vi "RGB_MNIST_PMT_sub.vi"(1 "pixel size":sgl=3.1, 2 "B_2D(28x28)":i32[][](array[numeric])=[[0, 0, 0, 0, 0, 0, 0, 0, 0, 0, 0, 0, 0, 0, 0, 0, 0, 0, 0, 0, 0, 0, 0, 0, 0, 0, 0, 0], [0, 0, 0, 0, 0, 0, 0, 0, 0, 0, 0, 1, 0, 0, 0, 0, 0, 0, 0, 0, 0, 0, 0, 0, 0, 0, 0, 0], [0, 0, 0, 0, 0, 0, 0, 0, 0, 0, 0, 3, 2, 0, 0, 0, 0, 0, 0, 0, 0, 0, 0, 0, 0, 0, 0, 0], [0, 0, 0, 0, 0, 0, 0, 6, 23, 26, 13, 4, 1, 0, 9, 27, 34, 24, 5, 0, 0, 0, 0, 0, 0, 0, 0, 0], [0, 0, 0, 0, 0, 0, 15, 47, 55, 55, 51, 40, 9, 7, 46, 57, 50, 16, 1, 0, 0, 0, 0, 0, 0, 0, 0, 0], [0, 0, 0, 0, 0, 12, 50, 57, 55, 57, 60, 63, 30, 30, 62, 82, 84, 72, 54, 20, 2, 0, 0, 0, 0, 0, 0, 0], [0, 0, 0, 0, 4, 44, 56, 54, 66, 89, 117, 131, 124, 100, 123, 137, 137, 138, 140, 138, 90, 26, 0, 0, 0, 0, 0, 0], [0, 0, 0, 0, 29, 55, 60, 91, 126, 139, 137, 136, 136, 136, 134, 133, 136, 137, 140, 142, 147, 131, 46, 0, 0, 0, 0, 0], [0, 0, 0, 10, 47, 62, 110, 151, 149, 145, 143, 143, 142, 139, 138, 136, 135, 137, 141, 144, 146, 150, 137, 36, 0, 0, 0, 0], [0, 0, 0, 27, 47, 104, 163, 161, 156, 155, 152, 150, 149, 146, 145, 140, 136, 137, 142, 144, 146, 150, 157, 109, 3, 0, 0, 0], [0, 0, 4, 14, 29, 139, 174, 168, 162, 162, 160, 158, 154, 153, 151, 144, 139, 138, 143, 144, 145, 148, 156, 141, 46, 0, 0, 0], [0, 0, 0, 0, 60, 167, 176, 170, 166, 165, 164, 162, 160, 156, 153, 150, 143, 140, 143, 144, 145, 147, 154, 155, 82, 0, 0, 0], [0, 0, 0, 0, 89, 185, 184, 175, 172, 168, 165, 163, 164, 161, 157, 153, 147, 142, 143, 144, 144, 146, 153, 160, 101, 0, 0, 0], [0, 0, 0, 0, 93, 191, 188, 180, 176, 170, 167, 168, 169, 165, 161, 156, 150, 143, 143, 144, 145, 147, 153, 159, 109, 6, 0, 0], [0, 0, 0, 0, 84, 186, 191, 185, 179, 173, 170, 170, 169, 166, 162, 157, 151, 144, 143, 144, 145, 148, 153, 159, 112, 11, 0, 0], [0, 0, 0, 0, 60, 178, 196, 190, 182, 176, 172, 171, 170, 167, 162, 157, 151, 144, 143, 144, 145, 149, 153, 159, 107, 4, 0, 0], [0, 0, 0, 0, 18, 165, 204, 193, 184, 177, 174, 171, 170, 167, 161, 158, 152, 143, 142, 144, 145, 149, 153, 159, 94, 0, 0, 0], [0, 0, 0, 0, 0, 121, 202, 195, 186, 179, 175, 171, 169, 167, 162, 158, 153, 144, 141, 144, 145, 149, 154, 150, 72, 0, 0, 0], [0, 0, 0, 0, 0, 38, 181, 200, 190, 181, 175, 172, 168, 166, 160, 158, 151, 142, 141, 144, 146, 149, 157, 135, 30, 0, 0, 0], [0, 0, 0, 0, 0, 0, 101, 204, 193, 182, 177, 172, 168, 165, 159, 157, 148, 138, 140, 144, 147, 149, 154, 90, 0, 0, 0, 0], [0, 0, 0, 0, 0, 0, 10, 121, 196, 184, 178, 171, 167, 162, 159, 156, 144, 137, 141, 143, 146, 149, 104, 14, 0, 0, 0, 0], [0, 0, 0, 0, 0, 0, 0, 11, 91, 176, 178, 171, 162, 157, 156, 148, 139, 138, 142, 145, 143, 86, 13, 0, 0, 0, 0, 0], [0, 0, 0, 0, 0, 0, 0, 0, 0, 41, 127, 162, 158, 152, 146, 141, 138, 138, 136, 116, 45, 2, 0, 0, 0, 0, 0, 0], [0, 0, 0, 0, 0, 0, 0, 0, 0, 0, 4, 49, 98, 121, 133, 144, 147, 121, 49, 5, 0, 0, 0, 0, 0, 0, 0, 0], [0, 0, 0, 0, 0, 0, 0, 0, 0, 0, 0, 0, 0, 17, 52, 83, 101, 55, 0, 0, 0, 0, 0, 0, 0, 0, 0, 0], [0, 0, 0, 0, 0, 0, 0, 0, 0, 0, 0, 0, 0, 0, 0, 1, 4, 2, 0, 0, 0, 0, 0, 0, 0, 0, 0, 0], [0, 0, 0, 0, 0, 0, 0, 0, 0, 0, 0, 0, 0, 0, 0, 0, 0, 0, 0, 0, 0, 0, 0, 0, 0, 0, 0, 0], [0, 0, 0, 0, 0, 0, 0, 0, 0, 0, 0, 0, 0, 0, 0, 0, 0, 0, 0, 0, 0, 0, 0, 0, 0, 0, 0, 0], [255, 0, 0, 0, 0, 0, 0, 0, 0, 0, 0, 0, 0, 0, 0, 0, 0, 0, 0, 0, 0, 0, 0, 0, 0, 0, 0, 0]], 3 "G_2D(28x28)":i32[][](array[numeric])=[[0, 0, 0, 0, 0, 0, 0, 0, 0, 0, 0, 0, 0, 0, 0, 0, 0, 0, 0, 0, 0, 0, 0, 0, 0, 0, 0, 0], [0, 0, 0, 0, 0, 0, 0, 0, 0, 0, 0, 1, 1, 0, 0, 0, 0, 0, 0, 0, 0, 0, 0, 0, 0, 0, 0, 0], [0, 0, 0, 0, 0, 0, 0, 0, 0, 0, 0, 6, 4, 0, 0, 0, 0, 0, 0, 0, 0, 0, 0, 0, 0, 0, 0, 0], [0, 0, 0, 0, 0, 0, 0, 13, 47, 51, 26, 8, 3, 0, 18, 54, 65, 45, 7, 0, 0, 0, 0, 0, 0, 0, 0, 0], [0, 0, 0, 0, 0, 0, 28, 90, 107, 109, 101, 75, 15, 14, 91, 112, 96, 30, 1, 0, 0, 0, 0, 0, 0, 0, 0, 0], [0, 0, 0, 0, 0, 23, 97, 113, 111, 110, 113, 117, 50, 55, 111, 117, 96, 71, 54, 20, 2, 0, 0, 0, 0, 0, 0, 0], [0, 0, 0, 0, 8, 85, 112, 109, 112, 119, 128, 132, 126, 112, 128, 137, 137, 138, 140, 138, 90, 26, 0, 0, 0, 0, 0, 0], [0, 0, 0, 0, 56, 109, 112, 122, 133, 137, 137, 136, 136, 136, 133, 134, 136, 137, 139, 142, 147, 131, 46, 0, 0, 0, 0, 0], [0, 0, 0, 18, 92, 116, 133, 149, 149, 145, 143, 143, 142, 139, 138, 136, 135, 137, 141, 143, 146, 150, 137, 36, 0, 0, 0, 0], [0, 0, 0, 53, 97, 128, 163, 161, 156, 155, 152, 150, 149, 146, 145, 141, 137, 137, 142, 144, 146, 150, 157, 109, 3, 0, 0, 0], [0, 0, 7, 28, 38, 140, 173, 168, 162, 162, 160, 158, 154, 153, 150, 144, 139, 138, 143, 144, 145, 148, 156, 141, 46, 0, 0, 0], [0, 0, 0, 0, 60, 167, 175, 170, 166, 165, 164, 162, 160, 156, 153, 150, 143, 140, 143, 144, 145, 148, 154, 155, 82, 0, 0, 0], [0, 0, 0, 0, 88, 184, 184, 176, 172, 168, 165, 163, 164, 161, 157, 153, 147, 142, 143, 144, 144, 147, 153, 160, 101, 0, 0, 0], [0, 0, 0, 0, 93, 190, 188, 180, 176, 171, 167, 168, 169, 165, 161, 156, 150, 143, 143, 144, 144, 147, 153, 159, 109, 6, 0, 0], [0, 0, 0, 0, 84, 186, 191, 185, 179, 173, 170, 170, 169, 166, 162, 157, 151, 144, 143, 144, 145, 148, 153, 159, 112, 11, 0, 0], [0, 0, 0, 0, 60, 177, 196, 190, 182, 176, 172, 171, 170, 167, 162, 157, 151, 144, 143, 144, 145, 149, 153, 159, 107, 4, 0, 0], [0, 0, 0, 0, 18, 165, 204, 193, 184, 177, 173, 171, 170, 167, 161, 158, 152, 145, 142, 144, 145, 149, 153, 159, 94, 0, 0, 0], [0, 0, 0, 0, 0, 121, 202, 195, 185, 178, 175, 172, 170, 167, 163, 159, 153, 144, 141, 144, 145, 150, 154, 150, 72, 0, 0, 0], [0, 0, 0, 0, 0, 38, 182, 200, 190, 181, 175, 172, 168, 166, 161, 159, 152, 142, 141, 144, 146, 149, 157, 135, 30, 0, 0, 0], [0, 0, 0, 0, 0, 0, 101, 204, 192, 182, 177, 172, 168, 165, 159, 158, 148, 138, 140, 144, 147, 149, 154, 90, 0, 0, 0, 0], [0, 0, 0, 0, 0, 0, 10, 122, 196, 184, 178, 171, 167, 162, 159, 156, 144, 137, 141, 143, 146, 149, 104, 14, 0, 0, 0, 0], [0, 0, 0, 0, 0, 0, 0, 11, 91, 176, 178, 169, 162, 157, 156, 148, 139, 139, 142, 144, 143, 86, 13, 0, 0, 0, 0, 0], [0, 0, 0, 0, 0, 0, 0, 0, 0, 42, 127, 162, 158, 152, 146, 141, 138, 138, 136, 116, 45, 2, 0, 0, 0, 0, 0, 0], [0, 0, 0, 0, 0, 0, 0, 0, 0, 0, 4, 50, 98, 121, 134, 144, 147, 121, 49, 5, 0, 0, 0, 0, 0, 0, 0, 0], [0, 0, 0, 0, 0, 0, 0, 0, 0, 0, 0, 0, 0, 17, 52, 83, 101, 55, 0, 0, 0, 0, 0, 0, 0, 0, 0, 0], [0, 0, 0, 0, 0, 0, 0, 0, 0, 0, 0, 0, 0, 0, 0, 1, 4, 2, 0, 0, 0, 0, 0, 0, 0, 0, 0, 0], [0, 0, 0, 0, 0, 0, 0, 0, 0, 0, 0, 0, 0, 0, 0, 0, 0, 0, 0, 0, 0, 0, 0, 0, 0, 0, 0, 0], [0, 0, 0, 0, 0, 0, 0, 0, 0, 0, 0, 0, 0, 0, 0, 0, 0, 0, 0, 0, 0, 0, 0, 0, 0, 0, 0, 0], [255, 0, 0, 0, 0, 0, 0, 0, 0, 0, 0, 0, 0, 0, 0, 0, 0, 0, 0, 0, 0, 0, 0, 0, 0, 0, 0, 0]], 4 "R_2D(28x28)":i32[][](array[numeric])=[[0, 0, 0, 0, 0, 0, 0, 0, 0, 0, 0, 0, 0, 0, 0, 0, 0, 0, 0, 0, 0, 0, 0, 0, 0, 0, 0, 0], [0, 0, 0, 0, 0, 0, 0, 0, 0, 0, 0, 3, 1, 0, 0, 0, 0, 0, 0, 0, 0, 0, 0, 0, 0, 0, 0, 0], [0, 0, 0, 0, 0, 0, 0, 0, 0, 0, 0, 14, 9, 0, 0, 0, 0, 0, 0, 0, 0, 0, 0, 0, 0, 0, 0, 0], [0, 0, 0, 0, 0, 0, 0, 12, 44, 49, 23, 15, 8, 0, 17, 51, 61, 42, 7, 0, 0, 0, 0, 0, 0, 0, 0, 0], [0, 0, 0, 0, 0, 0, 26, 84, 100, 102, 93, 73, 19, 13, 85, 104, 89, 27, 1, 0, 0, 0, 0, 0, 0, 0, 0, 0], [0, 0, 0, 0, 0, 21, 91, 106, 102, 104, 110, 115, 61, 55, 112, 147, 148, 128, 95, 35, 4, 0, 0, 0, 0, 0, 0, 0], [0, 0, 0, 0, 9, 80, 104, 102, 123, 166, 213, 237, 229, 181, 220, 244, 245, 247, 249, 241, 159, 45, 0, 0, 0, 0, 0, 0], [0, 0, 0, 0, 54, 100, 109, 163, 226, 250, 247, 245, 245, 248, 244, 243, 245, 245, 246, 249, 255, 226, 78, 0, 0, 0, 0, 0], [0, 0, 0, 18, 86, 112, 189, 252, 252, 249, 249, 250, 248, 247, 246, 245, 244, 246, 247, 249, 251, 255, 228, 60, 0, 0, 0, 0], [0, 0, 0, 50, 87, 171, 252, 255, 252, 253, 252, 252, 253, 251, 250, 248, 244, 245, 249, 250, 251, 253, 255, 182, 4, 0, 0, 0], [0, 0, 7, 26, 47, 212, 255, 255, 255, 254, 254, 254, 254, 255, 254, 251, 247, 246, 249, 250, 250, 252, 255, 232, 75, 0, 0, 0], [0, 0, 0, 0, 87, 237, 255, 255, 255, 254, 255, 254, 254, 255, 255, 253, 249, 248, 249, 250, 251, 252, 255, 255, 136, 0, 0, 0], [0, 0, 0, 0, 124, 252, 255, 255, 254, 254, 255, 255, 254, 255, 255, 255, 252, 248, 249, 250, 251, 251, 255, 255, 167, 0, 0, 0], [0, 0, 0, 0, 124, 252, 254, 254, 255, 255, 255, 255, 255, 254, 255, 255, 252, 247, 250, 250, 251, 252, 255, 255, 180, 10, 0, 0], [0, 0, 0, 0, 106, 241, 253, 254, 255, 255, 255, 255, 255, 255, 255, 253, 249, 248, 250, 250, 250, 253, 255, 255, 188, 19, 0, 0], [0, 0, 0, 0, 76, 228, 255, 255, 255, 255, 255, 255, 255, 255, 254, 250, 250, 250, 250, 250, 251, 253, 255, 255, 178, 7, 0, 0], [0, 0, 0, 0, 23, 208, 255, 255, 255, 255, 255, 255, 255, 254, 251, 253, 253, 249, 248, 250, 251, 253, 255, 255, 156, 0, 0, 0], [0, 0, 0, 0, 0, 152, 255, 255, 254, 255, 255, 255, 255, 254, 255, 255, 254, 249, 247, 250, 251, 254, 255, 250, 118, 0, 0, 0], [0, 0, 0, 0, 0, 48, 229, 255, 254, 254, 255, 255, 254, 255, 255, 255, 254, 248, 247, 249, 251, 253, 255, 221, 49, 0, 0, 0], [0, 0, 0, 0, 0, 0, 127, 253, 255, 254, 255, 254, 255, 255, 255, 255, 253, 246, 247, 250, 252, 253, 254, 150, 0, 0, 0, 0], [0, 0, 0, 0, 0, 0, 14, 154, 255, 255, 254, 255, 255, 255, 255, 255, 250, 245, 248, 249, 251, 255, 177, 23, 0, 0, 0, 0], [0, 0, 0, 0, 0, 0, 0, 13, 124, 245, 255, 255, 254, 255, 254, 251, 246, 247, 249, 250, 248, 149, 23, 0, 0, 0, 0, 0], [0, 0, 0, 0, 0, 0, 0, 0, 1, 60, 190, 250, 255, 255, 252, 248, 246, 246, 242, 202, 78, 5, 0, 0, 0, 0, 0, 0], [0, 0, 0, 0, 0, 0, 0, 0, 0, 0, 7, 80, 166, 211, 235, 254, 255, 215, 86, 8, 0, 0, 0, 0, 0, 0, 0, 0], [0, 0, 0, 0, 0, 0, 0, 0, 0, 0, 0, 0, 0, 29, 90, 146, 177, 95, 0, 0, 0, 0, 0, 0, 0, 0, 0, 0], [0, 0, 0, 0, 0, 0, 0, 0, 0, 0, 0, 0, 0, 0, 0, 1, 7, 2, 0, 0, 0, 0, 0, 0, 0, 0, 0, 0], [0, 0, 0, 0, 0, 0, 0, 0, 0, 0, 0, 0, 0, 0, 0, 0, 0, 0, 0, 0, 0, 0, 0, 0, 0, 0, 0, 0], [0, 0, 0, 0, 0, 0, 0, 0, 0, 0, 0, 0, 0, 0, 0, 0, 0, 0, 0, 0, 0, 0, 0, 0, 0, 0, 0, 0], [255, 0, 0, 0, 0, 0, 0, 0, 0, 0, 0, 0, 0, 0, 0, 0, 0, 0, 0, 0, 0, 0, 0, 0, 0, 0, 0, 0]]) -> (0 "picture":picture)   [LabVIEW 2021]
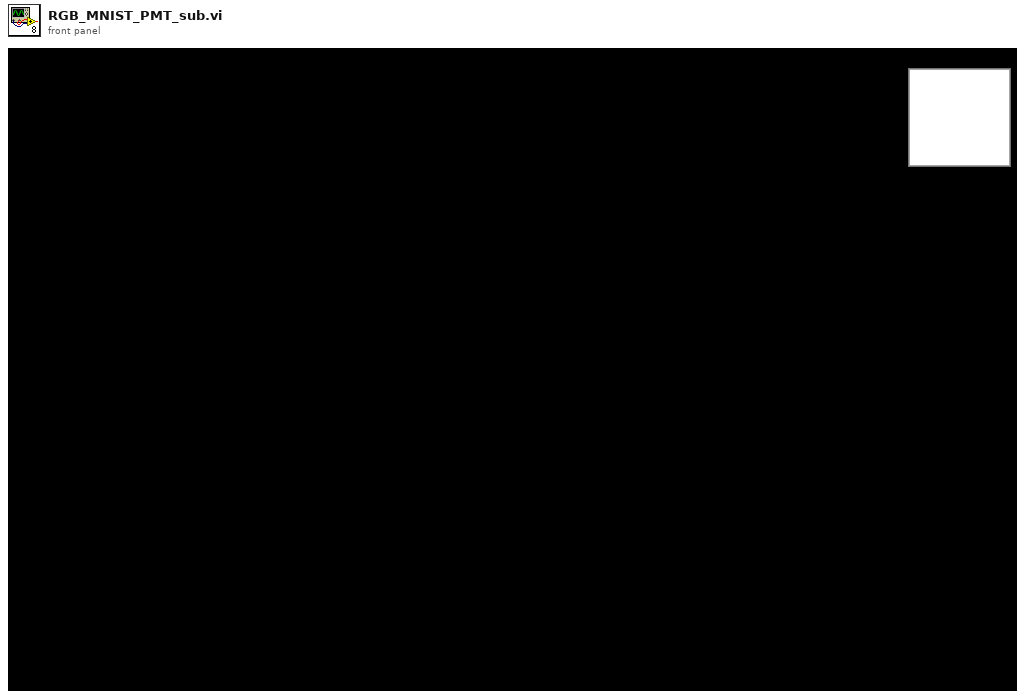
[diagram p1: front panel]
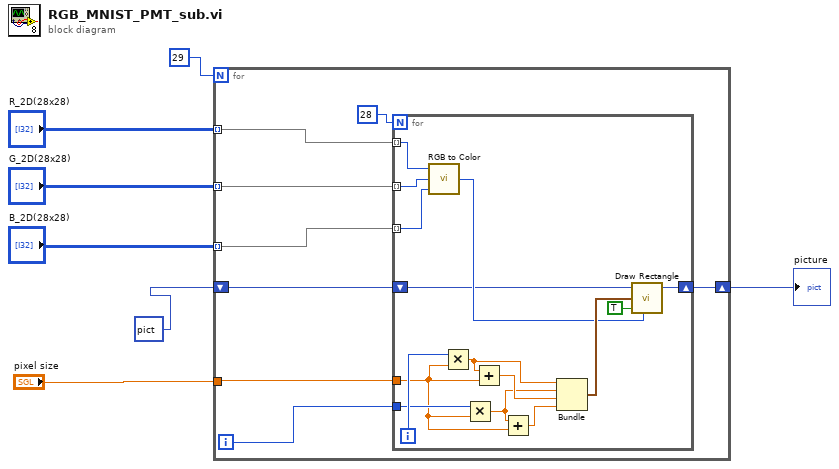
[diagram p0: block diagram]
diagram:
  n1 = for {
    N: 29 -> [_]
    tunnel: "R_2D(28x28)" -> [w15] mode=indexing
    tunnel: "G_2D(28x28)" -> [w14] mode=indexing
    tunnel: "B_2D(28x28)" -> [w13] mode=indexing
    tunnel: "pixel size" -> [w11]
    shift-right: [w9] -> w5
    shift-left: picture bytes[29792] ("picture 3") -> [w10]
    i -> [w12]
    n2 = for {
      N: 28 -> [_]
      tunnel: w15 -> [w29] mode=indexing
      tunnel: w14 -> [w28] mode=indexing
      tunnel: w13 -> [w27] mode=indexing
      tunnel: w12 -> [w21]
      tunnel: w11 -> [w20]
      shift-right: [w16] -> w9
      shift-left: w10 -> [w17]
      i -> [w22]
      n3 = call <vilib>:"RGB to Color.vi"("B"=w27, "G"=w28, "R"=w29) -> ("Color"=w18:u32)
      n4 = Multiply(x=w22, y=w20) -> (x*y=w26:sgl)
      n5 = Multiply(x=w21, y=w20) -> (x*y=w24:sgl)
      n6 = Add(x=w26, y=w20) -> (x+y=w25:sgl)
      n7 = Add(x=w24, y=w20) -> (x+y=w23:sgl)
      n8 = Bundle(w26, w24, w25, w23) -> (w19:cluster{sgl, sgl, sgl, sgl})  [unwired: 1 in]
      n9 = call <vilib>:"Draw Rectangle.vi"("picture"=w17, "rect"=w19, "fill?(F)"=TRUE, "color(black)"=w18) -> ("new picture"=w16:picture)  [unwired: 5 in]
    }
  }
  "picture" <- w5
